vi "Opgave 10 Dokumentation.vi"(8 "Numeric 2":dbl=2.0, 9 "Numeric":dbl=2.0, 11 "Enum":enum16{"Volumen", "Areal"}(ring)) -> (0 "Numeric 3":dbl)   [LabVIEW 2019]
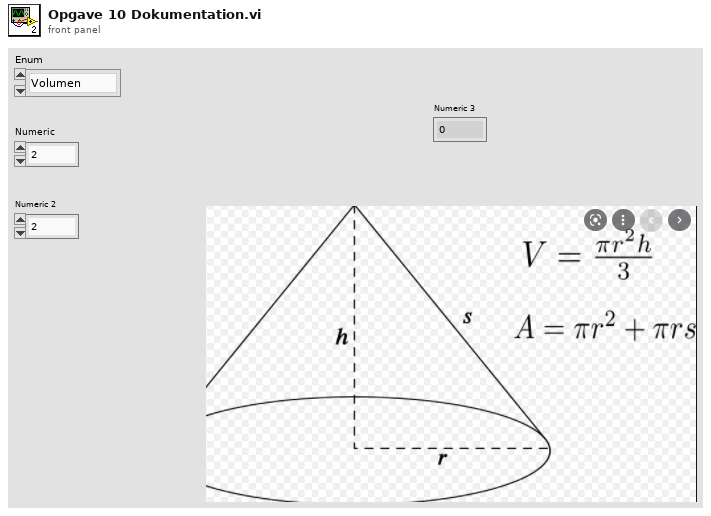
[diagram p1: front panel]
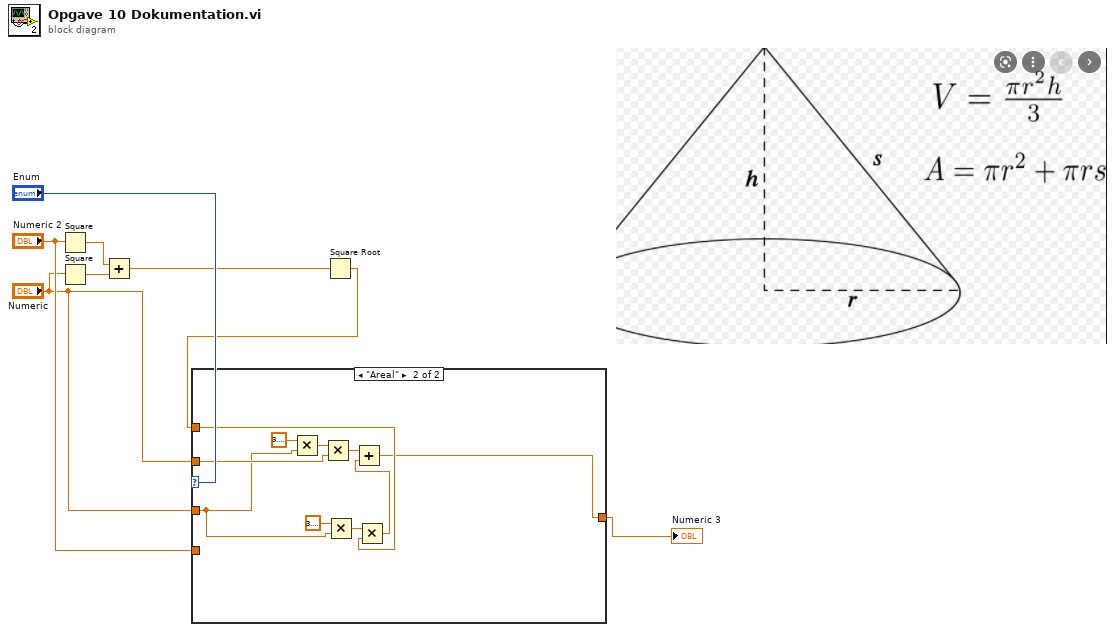
[diagram p0: block diagram]
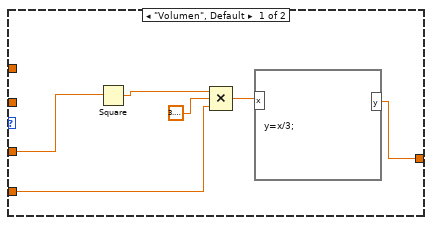
[diagram p2: hidden frame]
diagram:
  n1 = Square(x="Numeric 2") -> (x^2=w8:dbl)
  n2 = Square(x="Numeric") -> (x^2=w7:dbl)
  n3 = Add(x=w8, y=w7) -> (x+y=w4:dbl)
  n4 = Square Root(x=w4) -> (sqrt(x)=w2:dbl)
  n5 = case shown="\"Areal\"" "Enum" {
    tunnel: "Numeric" -> [_ w22]
    tunnel: "Numeric 2" -> [w12 _]
    tunnel: w2 -> [_ w17]
    tunnel: "Numeric" -> [w11 w19]
    tunnel: [w9 w15] -> w1
    frame "Volumen", Default {
      n6 = Square(x=w11) -> (x^2=w13:dbl)
      n7 = Compound Arithmetic op=MULTIPLY(w13, 3.141592653589793, w12) -> (w10:dbl)
      n8 = formula code="y=x/3;"("x"=w10) -> ("y"=w9:dbl)
    }
    frame "Areal" {
      n9 = Multiply(x=3.141592653589793, y=w19) -> (x*y=w23:dbl)
      n10 = Multiply(x=w23, y=w22) -> (x*y=w21:dbl)
      n11 = Multiply(x=3.141592653589793, y=w19) -> (x*y=w18:dbl)
      n12 = Multiply(x=w18, y=w17) -> (x*y=w16:dbl)
      n13 = Add(x=w21, y=w16) -> (x+y=w15:dbl)
    }
  }
  "Numeric 3" <- w1
